vi "TEST HI PRESSURE.vi"(8 "error in (no error)":errorcluster, 11 "Stand in":refnum<class "Stand.lvclass">) -> (0 "error out":errorcluster, 3 "Stand out":refnum<class "Stand.lvclass">)   [LabVIEW 2019, in "Stand.lvclass"]
uses:
  Stand.lvclass
  TypeDef/State HI_PERESS_TEST.ctl
  DO_class/DO.lvclass
  Sig_AI_class/Sig_AI.lvclass
  Sig_AO_class/Sig_AO.lvclass
  NeedleValve_class/NeedleValve.lvclass
  c1812564-f281-42cd-8b65-a881236ebb06.vi
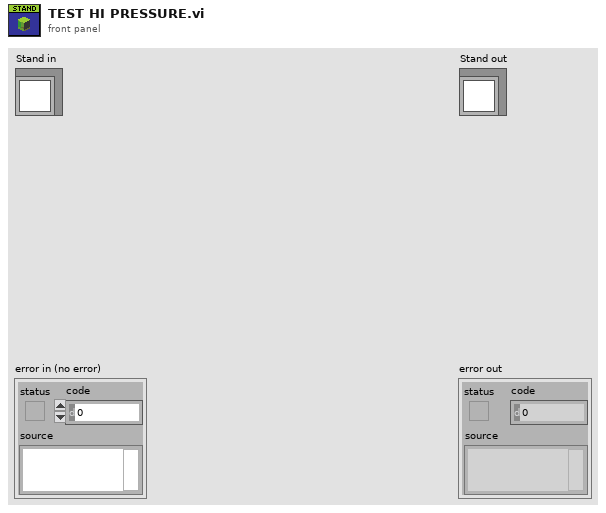
[diagram p1: front panel]
types:
  T1 = typedef "State HI_PERESS_TEST.ctl" = enum16{"NOT READY", "READY TO SUPPLY AIR", "PREPARE TO HI PRESS", "READY FOR HI PRESS", "CHECK DIRECTION", "INCREASING PRESSURE", "HOLDING", "PRESSURE RELEASE", "SOFT PRESSURE RELIEF", "ALARM"}
  T2 = typedef "AI_Data.ctl" = cluster{"Raw":dbl, "Scaled":dbl, "OutOfRangeMax":bool, "OutOfRangeMin":bool, "HIHI":bool, "HI":bool, "LO":bool, "LOLO":bool, "OutOfRangeMax_val":dbl, "OutOfRangeMin_val":dbl, "HIHI_val":dbl, "HI_val":dbl, "LO_val":dbl, "LOLO_val":dbl}
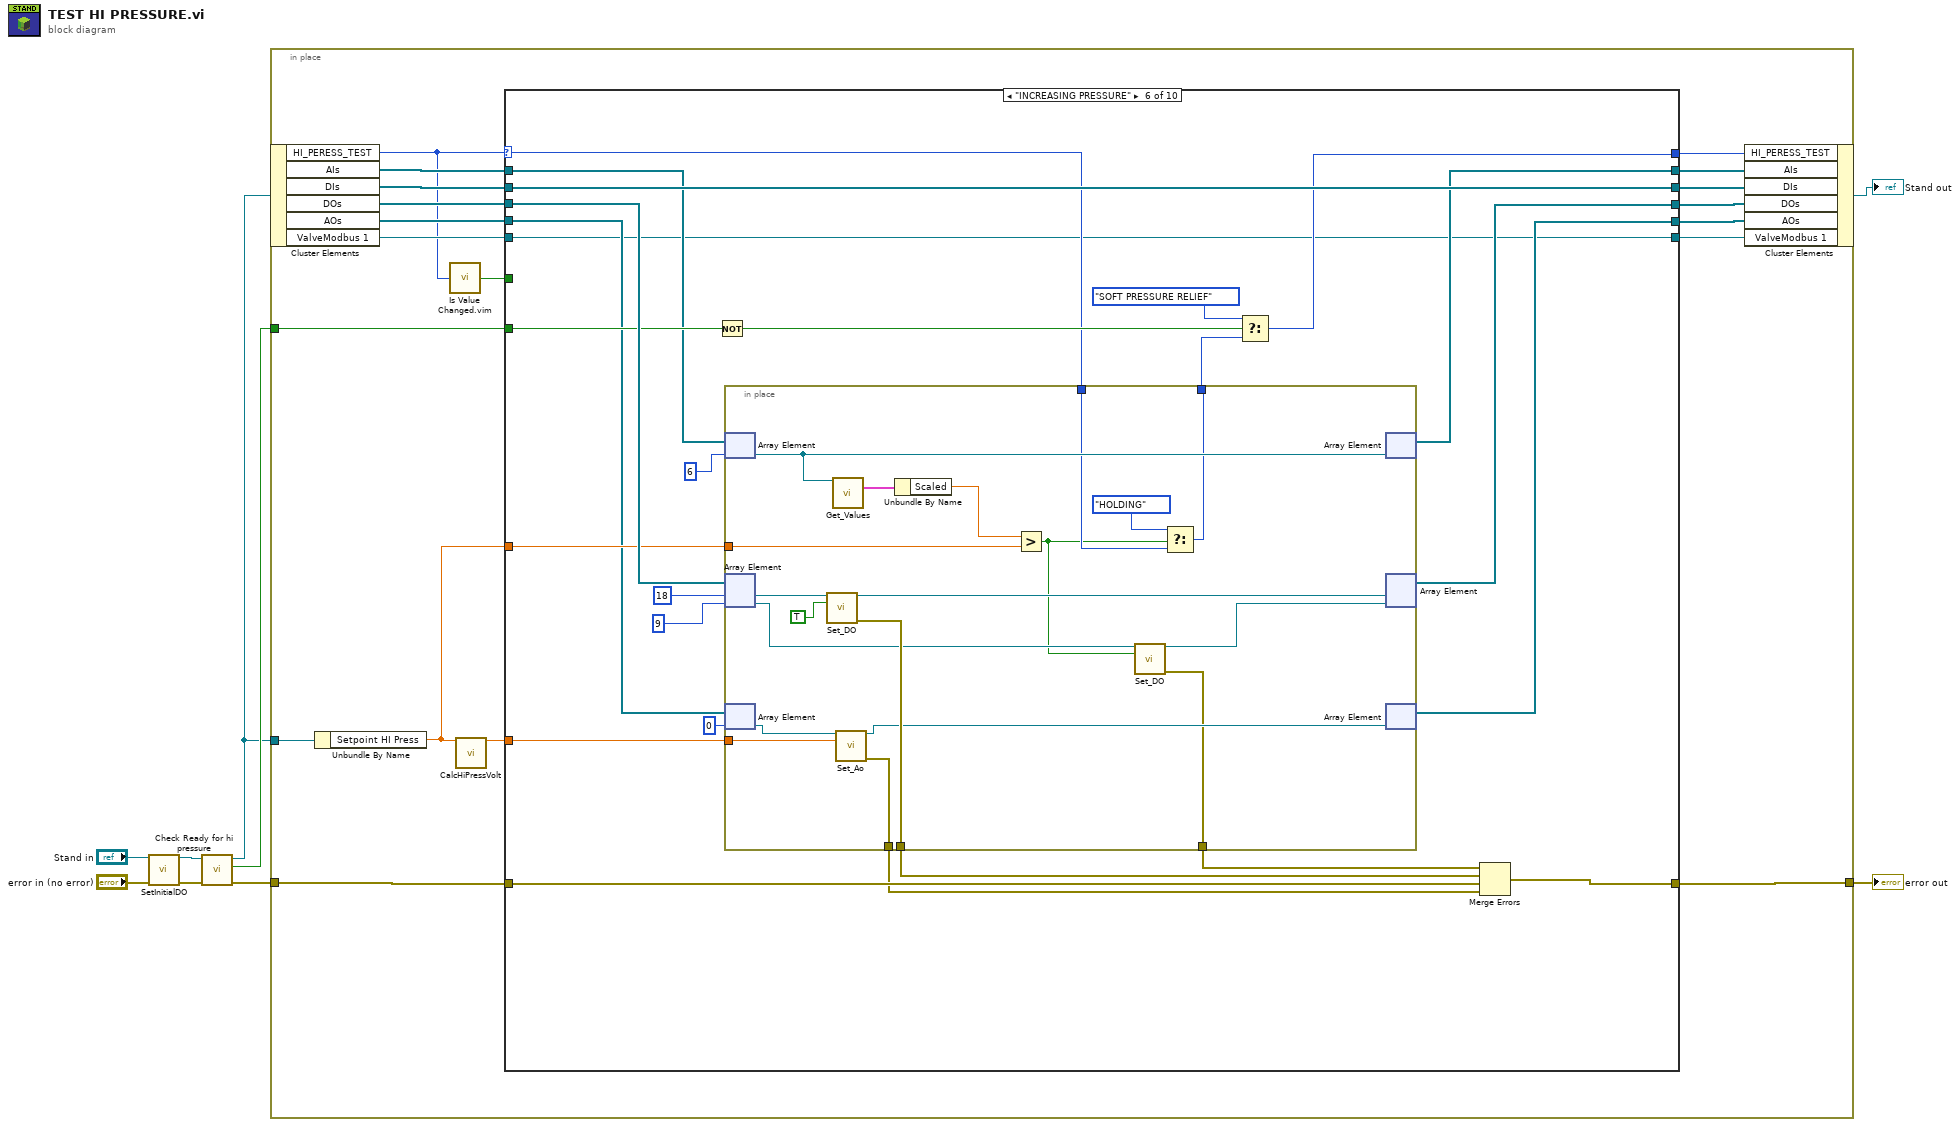
[diagram p0: block diagram]
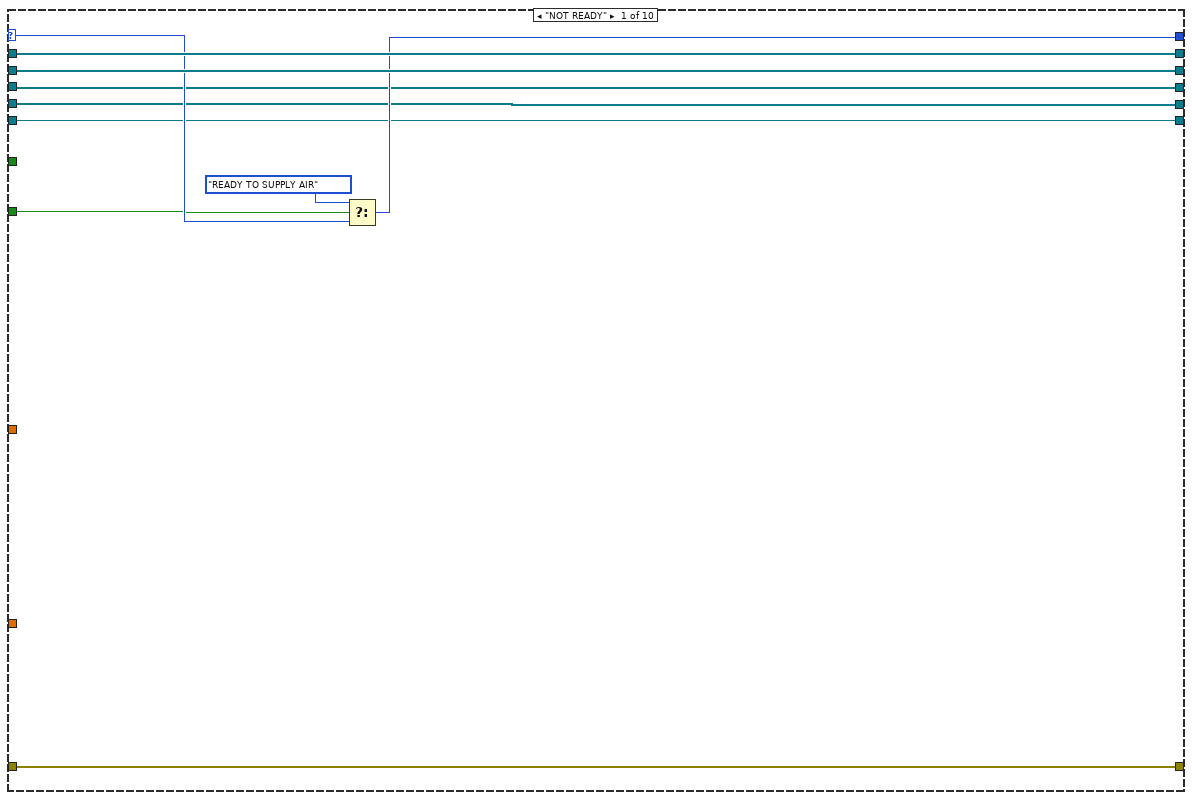
[diagram p2: hidden frame]
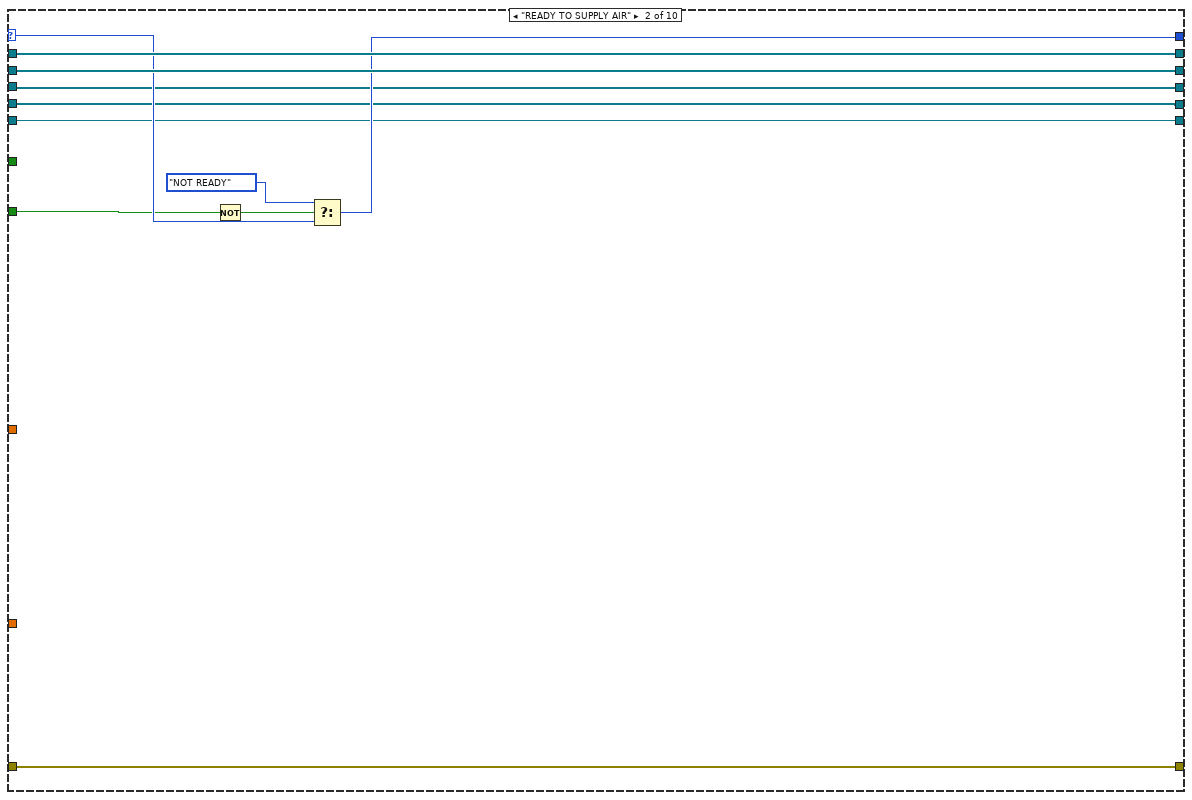
[diagram p3: hidden frame]
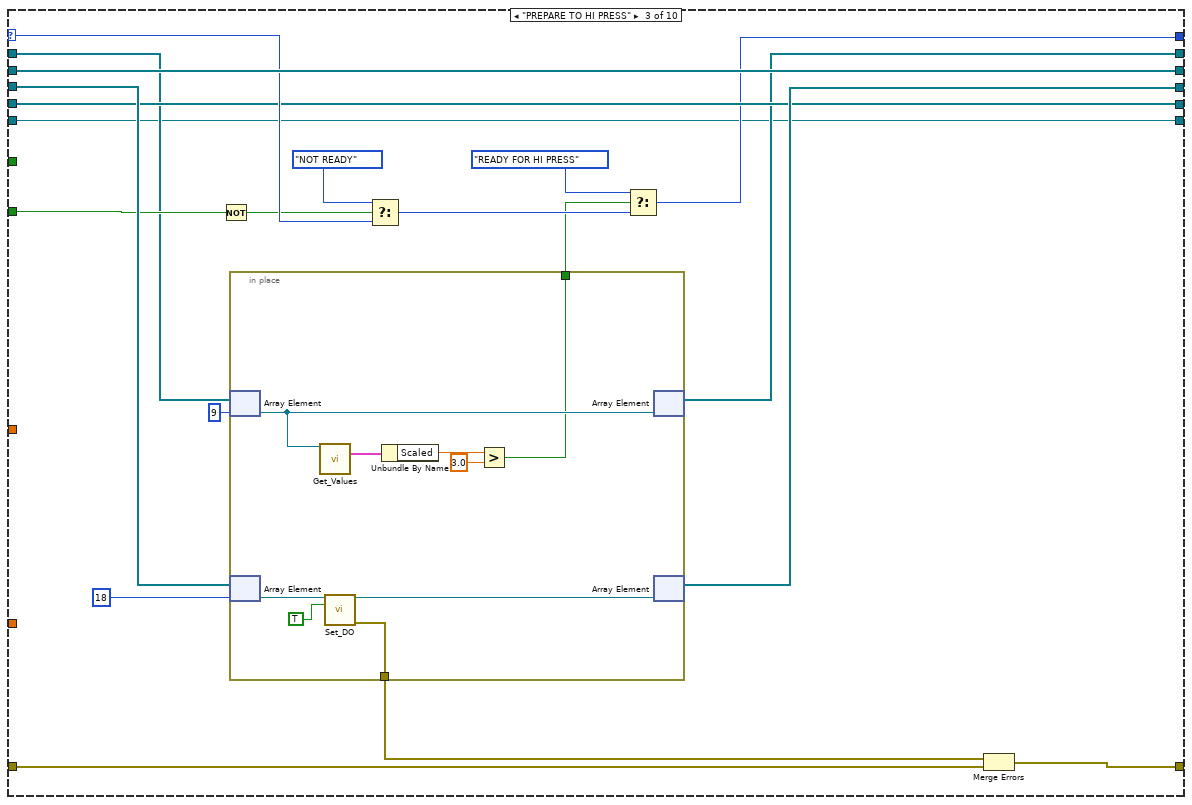
[diagram p4: hidden frame]
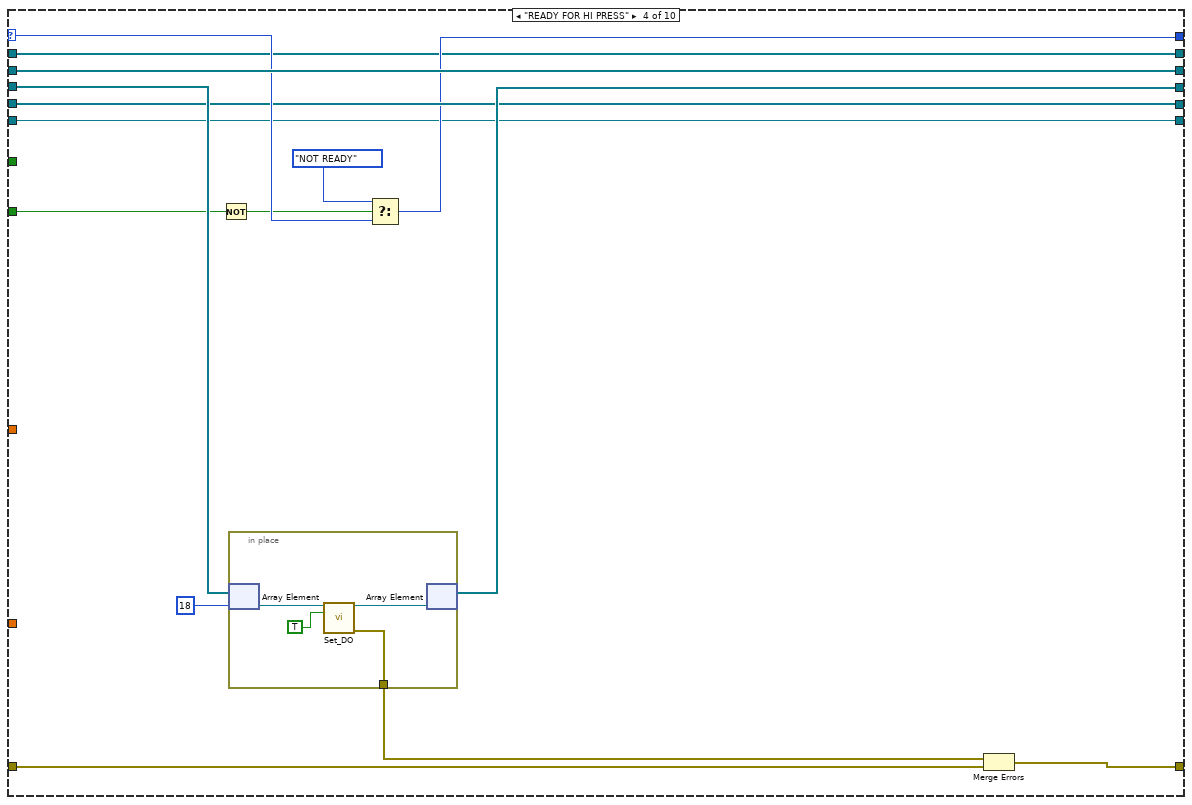
[diagram p5: hidden frame]
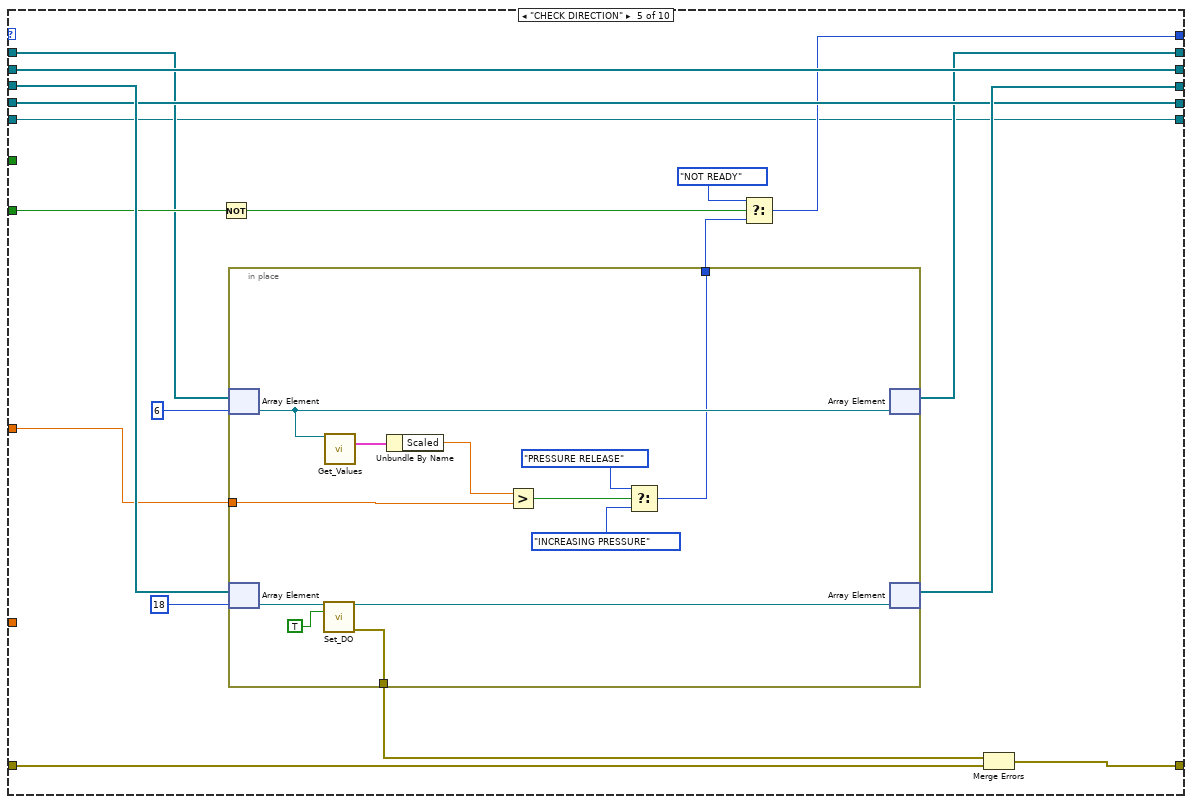
[diagram p6: hidden frame]
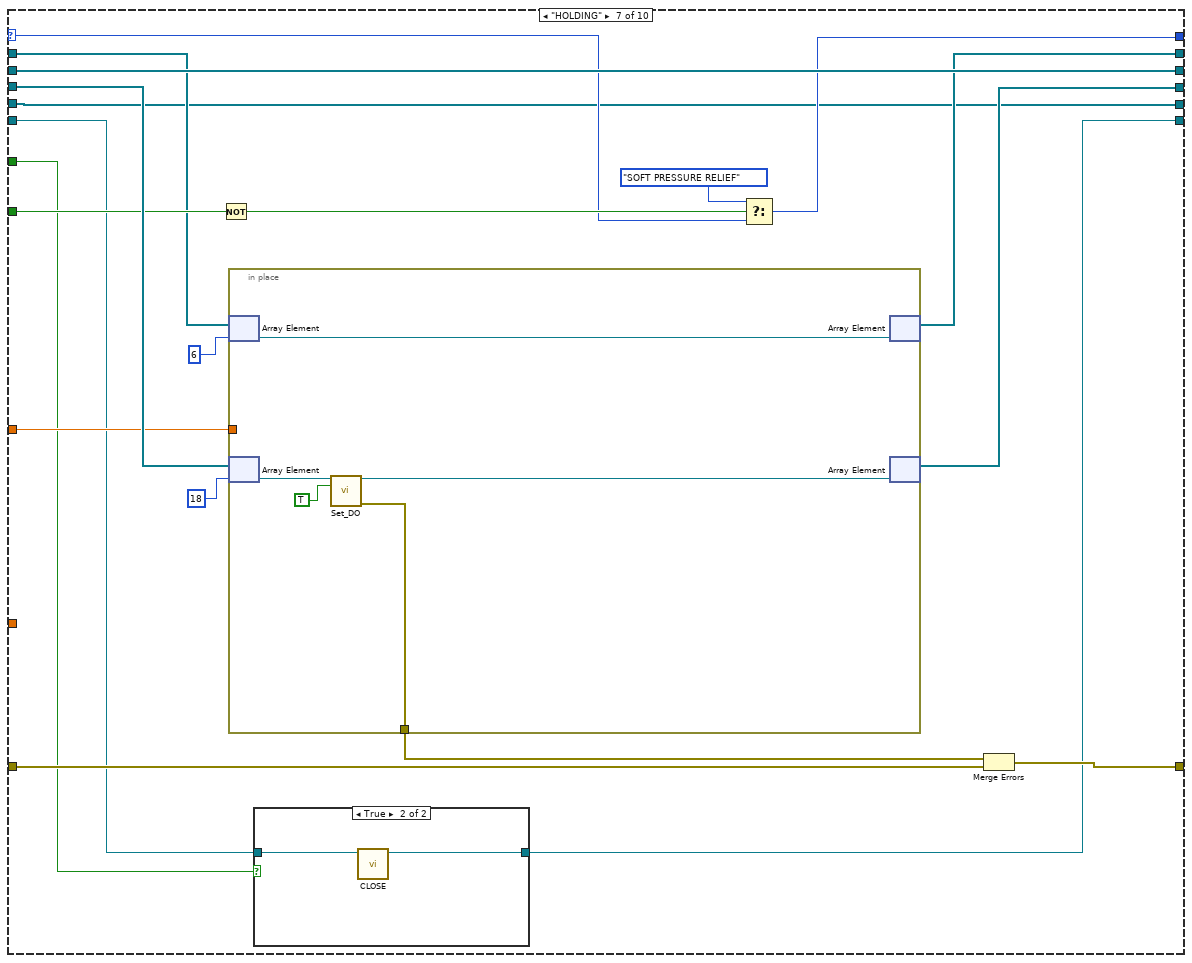
[diagram p7: hidden frame]
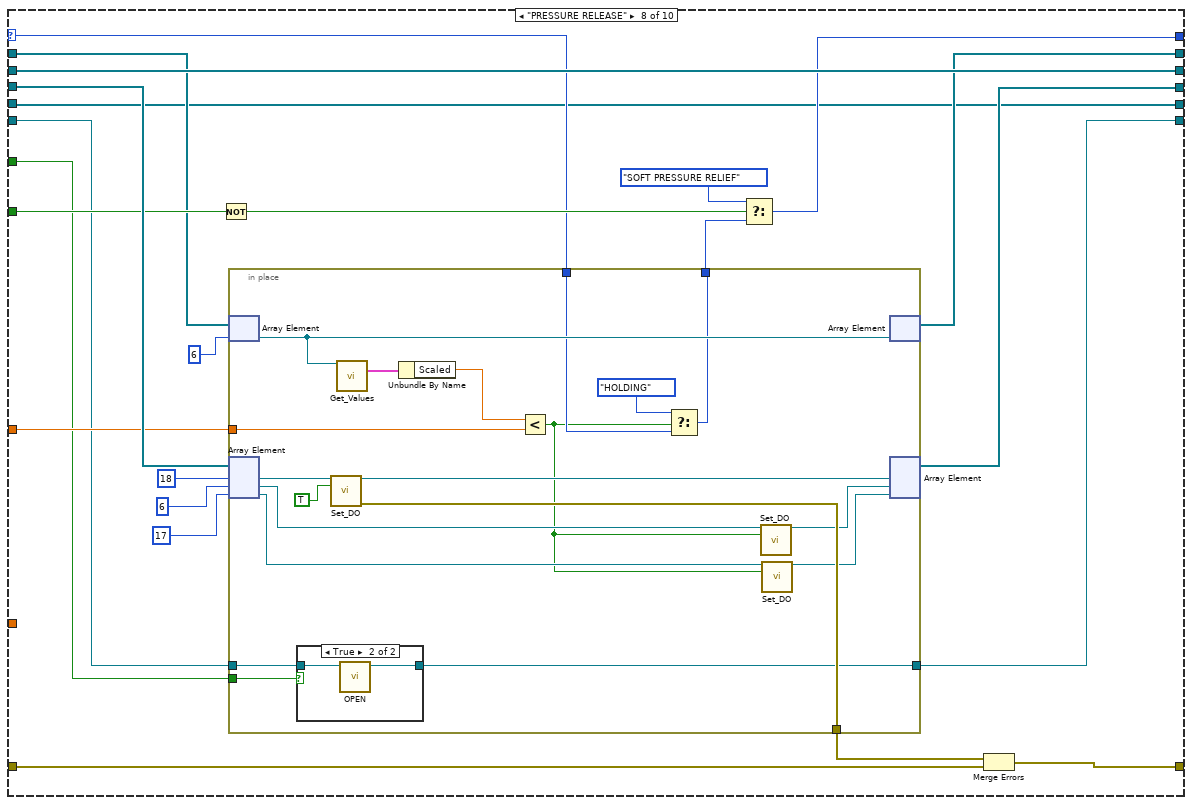
[diagram p9: hidden frame]
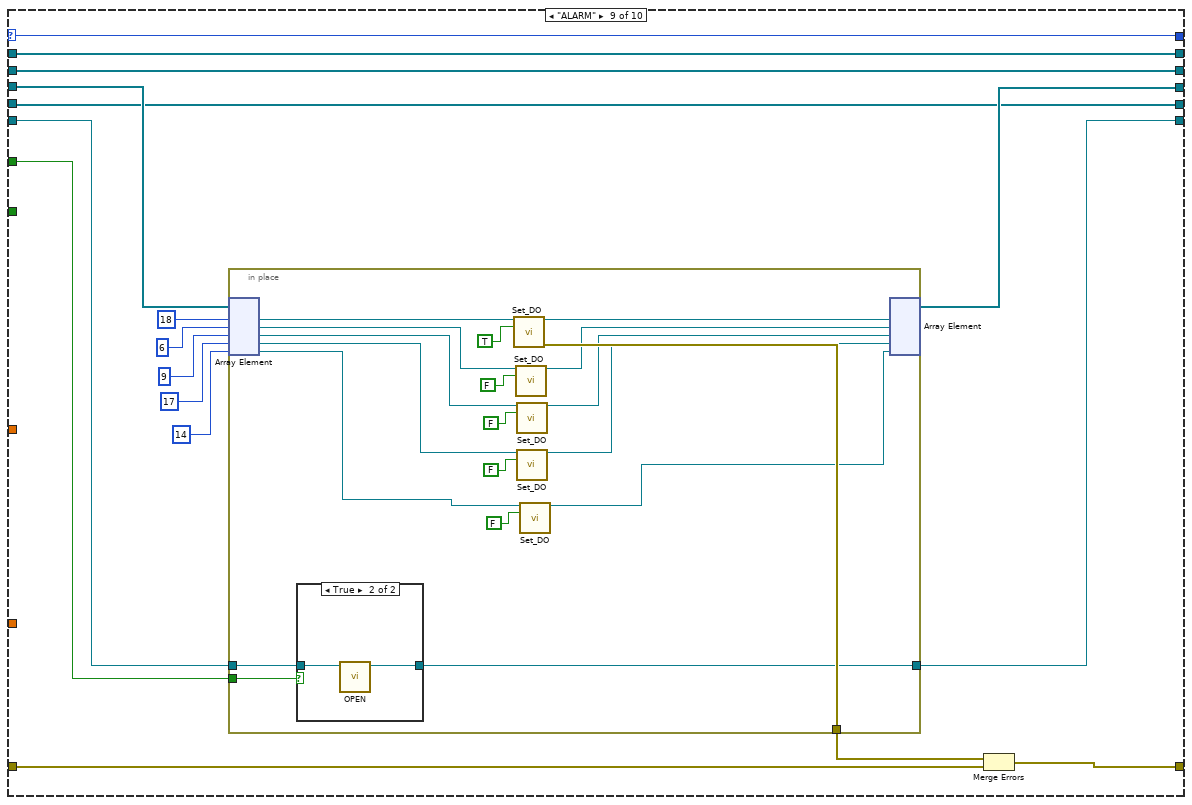
[diagram p11: hidden frame]
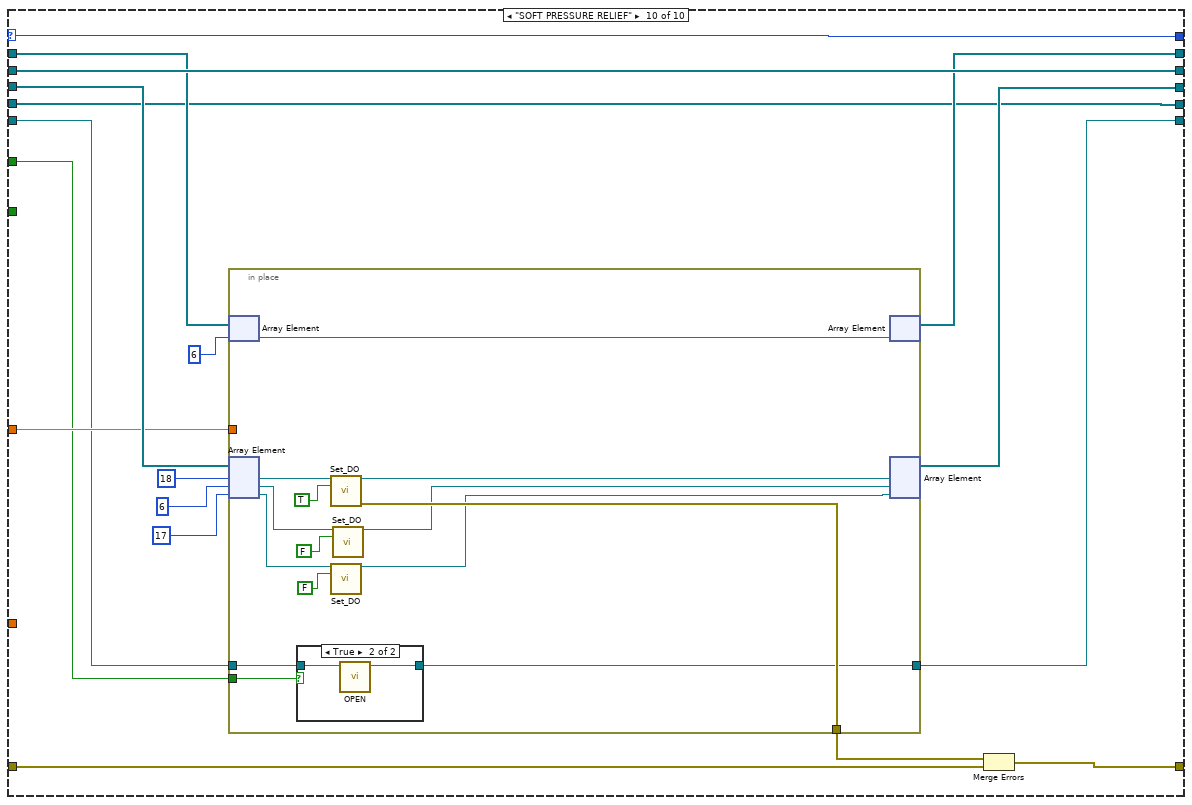
[diagram p13: hidden frame]
diagram:
  n1 = call "SetInitialDO.vi"("reference in"="Stand in", "error in"="error in (no error)") -> ("reference in 2"=w5:refnum<class "Stand.lvclass">, "error out"=w1:errorcluster)  [unwired: 12 in]
  n2 = call "Check Ready for hi pressure.vi"("error in (no error)"=w1, "Stand in"=w5) -> ("error out"=w3:errorcluster, "ready"=w7:bool, "Stand out"=w4:refnum<class "Stand.lvclass">)  [unwired: 7 in]
  n3 = in-place {
    in-place-border: [w28] -> w8
    in-place-border: w3 -> [w27]
    in-place-border: w4 -> [w17]
    in-place-border: w7 -> [w14]
    n4 = in-place-cluster #1(w4) -> ("HI_PERESS_TEST"=w11:T1, "AIs"=w24:refnum<class "Sig_AI.lvclass">[], "DIs"=w22:refnum<class "Sig_DI_Simple.lvclass">[], "DOs"=w20:refnum<class "DO.lvclass">[], "AOs"=w18:refnum<class "Sig_AO.lvclass">[], "ValveModbus 1"=w13:refnum<class "NeedleValve.lvclass">)
    n5 = Unbundle By Name(w17) -> ("Setpoint HI Press"=w15:dbl)
    n6 = call "Is Value Changed.vim"("value"=w11) -> ("changed or first call?"=w10:bool)
    n7 = call "CalcHiPressVolt.vi"("Setpoint HI Press"=w15) -> ("Numeric"=w16:dbl)  [unwired: 14 in]
    n8 = case shown="\"INCREASING PRESSURE\"" w11 {
      selector: w11 -> [w35 w46 w67 w91 _ w131 w176 w205 w248 w285]
      tunnel: [w38 w49 w63 w87 w110 w147 w186 w217 w257 w297] -> w28
      tunnel: w27 -> [w38 w49 w69 w93 w115 w152 w191 w222 w261 w301]
      tunnel: [w34 w45 w51 w81 w99 w137 w177 w207 w248 w285] -> w26
      tunnel: [w37 w48 w56 w80 w103 w141 w180 w211 w246 w293] -> w25
      tunnel: w24 -> [w37 w48 w57 w80 w104 w142 w181 w212 w246 w294]
      tunnel: [w36 w47 w68 w92 w114 w151 w190 w221 w260 w300] -> w23
      tunnel: w22 -> [w36 w47 w68 w92 w114 w151 w190 w221 w260 w300]
      tunnel: [w31 w41 w62 w86 w109 w146 w185 w216 w256 w296] -> w21
      tunnel: w20 -> [w31 w41 w65 w89 w112 w149 w188 w219 w259 w299]
      tunnel: [w30 w40 w59 w83 w106 w130 w172 w200 w249 w284] -> w19
      tunnel: w18 -> [w30 w40 w59 w83 w106 w135 w172 w200 w249 w284]
      tunnel: w16 -> [_ _ _ _ _ w134 _ _ _ _]
      tunnel: w15 -> [_ _ _ _ w101 w139 w178 w209 _ w291]
      tunnel: w14 -> [w32 w43 w61 w85 w108 w145 w184 w215 _ _]
      tunnel: w13 -> [w29 w39 w50 w79 w98 w129 w175 w203 w252 w288]
      tunnel: [w29 w39 w50 w79 w98 w129 w173 w202 w251 w287] -> w12
      tunnel: w10 -> [_ _ _ _ _ _ w174 w201 w250 w286]
      frame "NOT READY" {
        n9 = Select(t=State_HI_PERESS_TEST."READY TO SUPPLY AIR", s=w32, f=w35) -> (s? t:f=w34:T1)
      }
      frame "READY TO SUPPLY AIR" {
        n10 = Not(x=w43) -> (.not. x?=w42:bool)
        n11 = Select(t=State_HI_PERESS_TEST."NOT READY", s=w42, f=w46) -> (s? t:f=w45:T1)
      }
      frame "PREPARE TO HI PRESS" {
        n12 = Not(x=w61) -> (.not. x?=w60:bool)
        n13 = in-place {
          in-place-border: [w75] -> w58
          in-place-border: [w70] -> w52
          n14 = in-place-array #2(w57, 9) -> (w74:refnum<class "Sig_AI.lvclass">)
          n15 = in-place-array #3(w65, 18) -> (w78:refnum<class "DO.lvclass">)
          n16 = call "Get_Values.vi"("reference in"=w74) -> ("Data"=w73:T2)  [unwired: 13 in, 1 out]
          n17 = call "Set_DO.vi"("reference in"=w78, "DO"=TRUE) -> ("reference out"=w77:refnum<class "DO.lvclass">, "error out"=w75:errorcluster)  [unwired: 12 in]
          n18 = Unbundle By Name(w73) -> ("Scaled"=w72:dbl)
          n19 = Greater?(x=w72, y=3.0) -> (0:w70:bool)
          n20 = in-place-array #2(w74) -> (w56:refnum<class "Sig_AI.lvclass">[])  [unwired: 1 out]
          n21 = in-place-array #3(w77) -> (w62:refnum<class "DO.lvclass">[])  [unwired: 1 out]
        }
        n22 = Select(t=State_HI_PERESS_TEST."NOT READY", s=w60, f=w67) -> (s? t:f=w54:T1)
        n23 = Select(t=State_HI_PERESS_TEST."READY FOR HI PRESS", s=w52, f=w54) -> (s? t:f=w51:T1)
        n24 = Merge Errors(w58, w69) -> (w63:errorcluster)
      }
      frame "READY FOR HI PRESS" {
        n25 = Not(x=w85) -> (.not. x?=w84:bool)
        n26 = in-place {
          in-place-border: [w94] -> w82
          n27 = in-place-array #4(w89, 18) -> (w97:refnum<class "DO.lvclass">)
          n28 = call "Set_DO.vi"("reference in"=w97, "DO"=TRUE) -> ("reference out"=w96:refnum<class "DO.lvclass">, "error out"=w94:errorcluster)  [unwired: 12 in]
          n29 = in-place-array #4(w96) -> (w86:refnum<class "DO.lvclass">[])  [unwired: 1 out]
        }
        n30 = Select(t=State_HI_PERESS_TEST."NOT READY", s=w84, f=w91) -> (s? t:f=w81:T1)
        n31 = Merge Errors(w82, w93) -> (w87:errorcluster)
      }
      frame "CHECK DIRECTION" {
        n32 = Not(x=w108) -> (.not. x?=w107:bool)
        n33 = in-place {
          in-place-border: [w124] -> w105
          in-place-border: w101 -> [w120]
          in-place-border: [w116] -> w100
          n34 = in-place-array #5(w104, 6) -> (w121:refnum<class "Sig_AI.lvclass">)
          n35 = in-place-array #6(w112, 18) -> (w127:refnum<class "DO.lvclass">)
          n36 = call "Set_DO.vi"("reference in"=w127, "DO"=TRUE) -> ("reference out"=w126:refnum<class "DO.lvclass">, "error out"=w124:errorcluster)  [unwired: 12 in]
          n37 = call "Get_Values.vi"("reference in"=w121) -> ("Data"=w123:T2)  [unwired: 13 in, 1 out]
          n38 = Unbundle By Name(w123) -> ("Scaled"=w122:dbl)
          n39 = Greater?(x=w122, y=w120) -> (0:w119:bool)
          n40 = Select(t=State_HI_PERESS_TEST."PRESSURE RELEASE", s=w119, f=State_HI_PERESS_TEST."INCREASING PRESSURE" ("t")) -> (s? t:f=w116:T1)
          n41 = in-place-array #5(w121) -> (w103:refnum<class "Sig_AI.lvclass">[])  [unwired: 1 out]
          n42 = in-place-array #6(w126) -> (w109:refnum<class "DO.lvclass">[])  [unwired: 1 out]
        }
        n43 = Select(t=State_HI_PERESS_TEST."NOT READY", s=w107, f=w100) -> (s? t:f=w99:T1)
        n44 = Merge Errors(w105, w115) -> (w110:errorcluster)
      }
      frame "INCREASING PRESSURE" {
        n45 = Not(x=w145) -> (.not. x?=w144:bool)
        n46 = in-place {
          in-place-border: [w168] -> w143
          in-place-border: w139 -> [w164]
          in-place-border: [w156] -> w138
          in-place-border: w134 -> [w161]
          in-place-border: [w159] -> w132
          in-place-border: w131 -> [w158]
          in-place-border: [w155] -> w128
          n47 = in-place-array #7(w142, 6) -> (w165:refnum<class "Sig_AI.lvclass">)
          n48 = in-place-array #8(w149, 18, 9) -> (w171:refnum<class "DO.lvclass">, w163:refnum<class "DO.lvclass">)
          n49 = in-place-array #9(w135, 0) -> (w162:refnum<class "Sig_AO.lvclass">)
          n50 = call "Set_DO.vi"("reference in"=w171, "DO"=TRUE) -> ("reference out"=w170:refnum<class "DO.lvclass">, "error out"=w168:errorcluster)  [unwired: 12 in]
          n51 = call "Get_Values.vi"("reference in"=w165) -> ("Data"=w167:T2)  [unwired: 13 in, 1 out]
          n52 = call "Set_Ao.vi"("reference in"=w162, "AO"=w161) -> ("reference out"=w160:refnum<class "Sig_AO.lvclass">, "error out"=w159:errorcluster)  [unwired: 12 in]
          n53 = Unbundle By Name(w167) -> ("Scaled"=w166:dbl)
          n54 = Greater?(x=w166, y=w164) -> (0:w154:bool)
          n55 = call "Set_DO.vi"("reference in"=w163, "DO"=w154) -> ("reference out"=w153:refnum<class "DO.lvclass">, "error out"=w155:errorcluster)  [unwired: 12 in]
          n56 = Select(t=State_HI_PERESS_TEST."HOLDING", s=w154, f=w158) -> (s? t:f=w156:T1)
          n57 = in-place-array #7(w165) -> (w141:refnum<class "Sig_AI.lvclass">[])  [unwired: 1 out]
          n58 = in-place-array #8(w170, w153) -> (w146:refnum<class "DO.lvclass">[])  [unwired: 2 out]
          n59 = in-place-array #9(w160) -> (w130:refnum<class "Sig_AO.lvclass">[])  [unwired: 1 out]
        }
        n60 = Select(t=State_HI_PERESS_TEST."SOFT PRESSURE RELIEF", s=w144, f=w138) -> (s? t:f=w137:T1)
        n61 = Merge Errors(w128, w143, w152, w132) -> (w147:errorcluster)
      }
      frame "HOLDING" {
        n62 = Not(x=w184) -> (.not. x?=w183:bool)
        n63 = in-place {
          in-place-border: [w196] -> w182
          in-place-border: w178 -> [_]
          n64 = in-place-array #10(w181, 6) -> (w195:refnum<class "Sig_AI.lvclass">)
          n65 = in-place-array #11(w188, 18) -> (w199:refnum<class "DO.lvclass">)
          n66 = call "Set_DO.vi"("reference in"=w199, "DO"=TRUE) -> ("reference out"=w198:refnum<class "DO.lvclass">, "error out"=w196:errorcluster)  [unwired: 12 in]
          n67 = in-place-array #10(w195) -> (w180:refnum<class "Sig_AI.lvclass">[])  [unwired: 1 out]
          n68 = in-place-array #11(w198) -> (w185:refnum<class "DO.lvclass">[])  [unwired: 1 out]
        }
        n69 = case shown="True" w174 {
          tunnel: w175 -> [w192 w194]
          tunnel: [w192 w193] -> w173
          frame False {
          }
          frame True {
            n70 = call "CLOSE.vi"("Pump_1AI_1DO_2DI in"=w194) -> ("Pump_1AI_1DO_2DI out"=w193:refnum<class "NeedleValve.lvclass">)  [unwired: 10 in]
          }
        }
        n71 = Select(t=State_HI_PERESS_TEST."SOFT PRESSURE RELIEF", s=w183, f=w176) -> (s? t:f=w177:T1)
        n72 = Merge Errors(w182, w191) -> (w186:errorcluster)
      }
      frame "PRESSURE RELEASE" {
        n73 = Not(x=w215) -> (.not. x?=w214:bool)
        n74 = in-place {
          in-place-border: [w238] -> w213
          in-place-border: w209 -> [w234]
          in-place-border: [w229] -> w208
          in-place-border: w205 -> [w231]
          in-place-border: w203 -> [w226]
          in-place-border: [w225] -> w202
          in-place-border: w201 -> [w224]
          n75 = in-place-array #12(w212, 6) -> (w235:refnum<class "Sig_AI.lvclass">)
          n76 = in-place-array #13(w219, 18, 6, 17) -> (w241:refnum<class "DO.lvclass">, w233:refnum<class "DO.lvclass">, w228:refnum<class "DO.lvclass">)
          n77 = case shown="True" w224 {
            tunnel: w226 -> [w242 w244]
            tunnel: [w242 w243] -> w225
            frame False {
            }
            frame True {
              n78 = call "OPEN.vi"("Pump_1AI_1DO_2DI in"=w244) -> ("Pump_1AI_1DO_2DI out"=w243:refnum<class "NeedleValve.lvclass">)  [unwired: 10 in]
            }
          }
          n79 = call "Set_DO.vi"("reference in"=w241, "DO"=TRUE) -> ("reference out"=w240:refnum<class "DO.lvclass">, "error out"=w238:errorcluster)  [unwired: 12 in]
          n80 = call "Get_Values.vi"("reference in"=w235) -> ("Data"=w237:T2)  [unwired: 13 in, 1 out]
          n81 = Unbundle By Name(w237) -> ("Scaled"=w236:dbl)
          n82 = Less?(x=w236, y=w234) -> (x < y?=w223:bool)
          n83 = Select(t=State_HI_PERESS_TEST."HOLDING", s=w223, f=w231) -> (s? t:f=w229:T1)
          n84 = call "Set_DO.vi"("reference in"=w233, "DO"=w223) -> ("reference out"=w232:refnum<class "DO.lvclass">)  [unwired: 12 in, 1 out]
          n85 = call "Set_DO.vi"("reference in"=w228, "DO"=w223) -> ("reference out"=w227:refnum<class "DO.lvclass">)  [unwired: 12 in, 1 out]
          n86 = in-place-array #12(w235) -> (w211:refnum<class "Sig_AI.lvclass">[])  [unwired: 1 out]
          n87 = in-place-array #13(w240, w232, w227) -> (w216:refnum<class "DO.lvclass">[])  [unwired: 3 out]
        }
        n88 = Select(t=State_HI_PERESS_TEST."SOFT PRESSURE RELIEF", s=w214, f=w208) -> (s? t:f=w207:T1)
        n89 = Merge Errors(w213, w222) -> (w217:errorcluster)
      }
      frame "ALARM" {
        n90 = in-place {
          in-place-border: [w277] -> w255
          in-place-border: w252 -> [w272]
          in-place-border: [w271] -> w251
          in-place-border: w250 -> [w270]
          n91 = in-place-array #14(w259, 18, 6, 9, 17, 14) -> (w280:refnum<class "DO.lvclass">, w276:refnum<class "DO.lvclass">, w274:refnum<class "DO.lvclass">, w266:refnum<class "DO.lvclass">, w263:refnum<class "DO.lvclass">)
          n92 = case shown="True" w270 {
            tunnel: w272 -> [w281 w283]
            tunnel: [w281 w282] -> w271
            frame False {
            }
            frame True {
              n93 = call "OPEN.vi"("Pump_1AI_1DO_2DI in"=w283) -> ("Pump_1AI_1DO_2DI out"=w282:refnum<class "NeedleValve.lvclass">)  [unwired: 10 in]
            }
          }
          n94 = call "Set_DO.vi"("reference in"=w280, "DO"=TRUE) -> ("reference out"=w279:refnum<class "DO.lvclass">, "error out"=w277:errorcluster)  [unwired: 12 in]
          n95 = call "Set_DO.vi"("reference in"=w276, "DO"=FALSE) -> ("reference out"=w275:refnum<class "DO.lvclass">)  [unwired: 12 in, 1 out]
          n96 = call "Set_DO.vi"("reference in"=w274, "DO"=FALSE) -> ("reference out"=w273:refnum<class "DO.lvclass">)  [unwired: 12 in, 1 out]
          n97 = call "Set_DO.vi"("reference in"=w266, "DO"=FALSE) -> ("reference out"=w265:refnum<class "DO.lvclass">)  [unwired: 12 in, 1 out]
          n98 = call "Set_DO.vi"("reference in"=w263, "DO"=FALSE) -> ("reference out"=w262:refnum<class "DO.lvclass">)  [unwired: 12 in, 1 out]
          n99 = in-place-array #14(w279, w275, w273, w265, w262) -> (w256:refnum<class "DO.lvclass">[])  [unwired: 5 out]
        }
        n100 = Merge Errors(w255, w261) -> (w257:errorcluster)
      }
      frame "SOFT PRESSURE RELIEF" {
        n101 = in-place {
          in-place-border: [w312] -> w295
          in-place-border: w291 -> [_]
          in-place-border: w288 -> [w304]
          in-place-border: [w303] -> w287
          in-place-border: w286 -> [w302]
          n102 = in-place-array #15(w294, 6) -> (w311:refnum<class "Sig_AI.lvclass">)
          n103 = in-place-array #16(w299, 18, 6, 17) -> (w315:refnum<class "DO.lvclass">, w309:refnum<class "DO.lvclass">, w306:refnum<class "DO.lvclass">)
          n104 = case shown="True" w302 {
            tunnel: w304 -> [w316 w318]
            tunnel: [w316 w317] -> w303
            frame False {
            }
            frame True {
              n105 = call "OPEN.vi"("Pump_1AI_1DO_2DI in"=w318) -> ("Pump_1AI_1DO_2DI out"=w317:refnum<class "NeedleValve.lvclass">)  [unwired: 10 in]
            }
          }
          n106 = call "Set_DO.vi"("reference in"=w315, "DO"=TRUE) -> ("reference out"=w314:refnum<class "DO.lvclass">, "error out"=w312:errorcluster)  [unwired: 12 in]
          n107 = call "Set_DO.vi"("reference in"=w306, "DO"=FALSE) -> ("reference out"=w305:refnum<class "DO.lvclass">)  [unwired: 12 in, 1 out]
          n108 = call "Set_DO.vi"("reference in"=w309, "DO"=FALSE) -> ("reference out"=w308:refnum<class "DO.lvclass">)  [unwired: 12 in, 1 out]
          n109 = in-place-array #15(w311) -> (w293:refnum<class "Sig_AI.lvclass">[])  [unwired: 1 out]
          n110 = in-place-array #16(w314, w308, w305) -> (w296:refnum<class "DO.lvclass">[])  [unwired: 3 out]
        }
        n111 = Merge Errors(w295, w301) -> (w297:errorcluster)
      }
    }
    n112 = in-place-cluster #1("HI_PERESS_TEST"=w26, "AIs"=w25, "DIs"=w23, "DOs"=w21, "AOs"=w19, "ValveModbus 1"=w12) -> (→"Stand out":refnum<class "Stand.lvclass">)
  }
  "error out" <- w8
